vi "closed_loop_arbitrary_binary_stim.vi"() -> ()   [LabVIEW 2014]
uses:
  <vilib>/vision/Measure.llb/Straight Edge Options.ctl
  <vilib>/vision/Measure.llb/Straight Edge Process.ctl
  <vilib>/Platform/TimedLoop/XDataNode/timing_clust.ctl
  <vilib>/Platform/TimedLoop/XDataNode/nitl_modes.ctl
  <vilib>/Platform/TimedLoop/XDataNode/wakeup.ctl
  <vilib>/vision/Measure.llb/Edge Options.ctl
  <vilib>/vision/Measure.llb/Edge Polarity.ctl
  <vilib>/DAQmx/create/channels.llb/DAQmx Create Channel (DO-Digital Output).vi
  <vilib>/DAQmx/write.llb/DAQmx Write (Digital Bool 1Line 1Point).vi
  <vilib>/gmath/statdist.llb/Uniform (Discrete) Random.vi
  <vilib>/DAQmx/create/channels.llb/DAQmx Create Channel (AO-Voltage-Basic).vi
  <vilib>/Platform/TimedLoop/TimeConversion.llb/rt-rel-time-to-milliseconds.vi
  <vilib>/DAQmx/write.llb/DAQmx Write (Analog DBL 1Chan 1Samp).vi
  <vilib>/DAQmx/create/channels.llb/DAQmx Create Channel (DI-Digital Input).vi
  <vilib>/DAQmx/read.llb/DAQmx Read (Digital Bool 1Line 1Point).vi
  <vilib>/platform/TimedLoop/XDataNode/XDataNode.xnode
  <vilib>/vision/driver/NI_Vision_Acquisition_Software.lvlib
  <vilib>/Platform/TimedLoop/XDataNode/XDNodeRunTimeDep.lvlib
  <vilib>/vision/NI_Vision_Development_Module.lvlib
  <vilib>/gmath/NI_Gmath.lvlib
panel:
  out "Slide 5":dbl(slide) scale=0.0..1.0
  out "Stim 4":i32
  in  "Stimulus Folder":path=path "C:/Users/nagellab/Documents/MATLAB/wind_pulses"
  in  "Stimulus Duration (s)":dbl=80.0
  out "Light History":i16(graph)
  out "Wind History":i16(graph)
  in  "Initial Orientation (for each trial)":dbl
  out "Light":bool=TRUE
  in  "Light Intensity (V)":dbl=3.9 format="%#_13g"
  in  "Wind Intensity (V)":dbl=3.1 format="%#_13g"
  out "Wind":bool=TRUE
  out "H0":dbl
  out "Slide 4":dbl(slide) scale=0.0..1.0
  out "Slide 3":dbl(slide) scale=0.0..1.0
  out "Slide 2":dbl(slide) scale=0.0..1.0
  out "Stim 3":i32
  out "Stim 2":i32
  out "Stim 1":i32
  in  "Reversed Tether?":bool=TRUE
  in  "R options":T1={"Number of Lines"=1, "Type"=enum."Best Edge Projection", "Min. Score"=10.0, "Max. Score"=1000.0, "Orientation"=-135.0, "Angle Range"=45.0, "Angle Tolerance"=1.0, "Step Size"=3, "Min. SNR (db)"=0.0, "Min. Points (%)"=25.0, "Hough Iterations"=3} {"Min. Points (%)" min=0.0 max=100.0; "Min. SNR (db)" min=0.0; "Max. Score" min=0.0 max=1024.0; "Min. Score" min=0.0 max=1024.0 step=1.0}
  in  "L options":T1={"Number of Lines"=1, "Type"=enum."Best Edge Projection", "Min. Score"=10.0, "Max. Score"=1000.0, "Orientation"=135.0, "Angle Range"=45.0, "Angle Tolerance"=1.0, "Step Size"=3, "Min. SNR (db)"=0.0, "Min. Points (%)"=25.0, "Hough Iterations"=3} {"Min. Points (%)" min=0.0 max=100.0; "Min. SNR (db)" min=0.0; "Max. Score" min=0.0 max=1024.0; "Min. Score" min=0.0 max=1024.0 step=1.0}
  out "Slide":dbl(slide) scale=0.0..1.0
  out "Motor Error":bool
  in  "Max steps/sample":dbl=6.0
  in  "Step Rate (Hz)":dbl=500.0
  out "Heading (deg)":dbl(graph)
  out "H":dbl format="%.4f"
  out "X (steps/sample)":dbl
  in  "Geneotype":string="w+ Canton-S"
  in  "Starvation Time (hrs)":string="1"
  in  "Age (DSE)":string="4"
  out "Trial End":bool
  in  "Trial Duration (s)":dbl=80.0
  out "Trial":i32 format="%#.3f"
  in  "Number of Trials":i32=12
  in  "Experiment name":string="E1"
  in  "Fly ID":string
  in  "L-R WBA Offset (deg)":dbl format="%#_13g"
  in  "deltaWBA Gain (g, unitless)":dbl=0.04 format="%.4f"
  out "L-R WBA":dbl
  out "deltaWBA":dbl format="%.4f"
  out "Scaled deltaWBA (deg)":dbl(graph)
  out "R WBA":dbl
  out "L WBA":dbl
  out "Image":T3(plugin-control)
  in  "Image Threshold":cluster{"Lower value":sgl, "Upper value":sgl}={"Lower value"=130.0, "Upper value"=255.0} {"Upper value" format="%.2f"; "Lower value" format="%.2f"}
  in  "Data Rate (Hz)":dbl=50.0
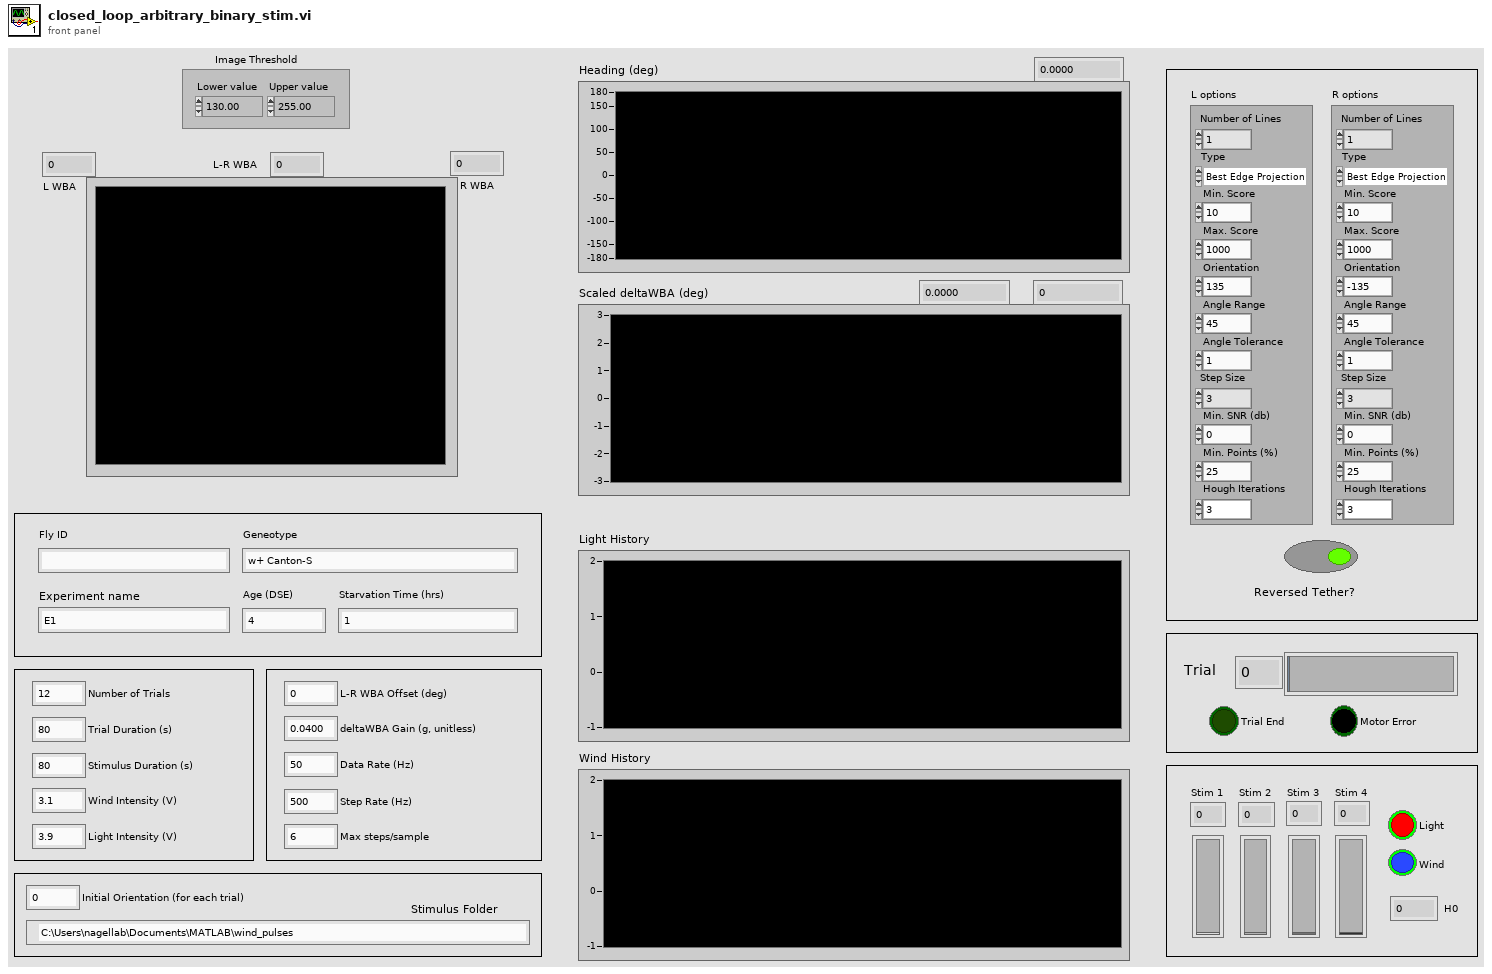
[diagram p1: front panel]
types:
  T1 = typedef "Straight Edge Options.ctl" = cluster{"Number of Lines":i32, "Type":T2, "Min. Score":dbl, "Max. Score":dbl, "Orientation":dbl, "Angle Range":dbl, "Angle Tolerance":dbl, "Step Size":u32, "Min. SNR (db)":dbl, "Min. Points (%)":dbl, "Hough Iterations":i32}
  T2 = typedef "Straight Edge Process.ctl" = enum32{"First Edge Rake", "Best Edge Rake", "Hough Edge Rake", "First Edge Projection", "Best Edge Projection"}
  T3 = typedef "IMAQ Image.ctl" = refnum<image>
  T4 = enum16{"open", "replace", "create", "open or create", "replace or create", "replace or create with confirmation"}
  T5 = typedef "IMAQdx.ctl" = refnum<k21>
  T6 = typedef "IMAQ Rectangle" = cluster{"Left":i32, "Top":i32, "Right":i32, "Bottom":i32, "Rotation":dbl}
  T7 = typedef "ROI Descriptor" = cluster{"Global Rectangle":i32[], "Contours":cluster{"ID":enum32{"External", "Internal"}, "Type":u32, "Coordinates":i32[]}[]}
  T8 = enum16{"big-endian, network order", "native, host order", "little-endian"}
  T9 = typedef "XDNodeRunTimeDep.lvlib/timing_clust.ctl" = cluster{"Expected End [f-1]":u64, "Actual End [f-1]":u64, "Finished Late? [f-1]":bool, "Expected End [i-1]":u64, "Actual End [i-1]":u64, "Finished Late? [i-1]":bool, "Expected Start [i]":u64, "Actual Start [i]":u64, "Expected Start [f]":u64, "Actual Start [f]":u64, "Source Name":string, "Structure Name":string, "Period":i64, "Deadline":i64, "Offset":i64, "Start":i64, "Priority":i32, "Timeout":i32, "Mode":T10, "Wakeup Reason":T11, "Error":errorcluster, "Source Type":string, "Secondary Source Type":string, "Global End Time":u64, "Global Start Time":u64, "Frame Duration":u64, "Iteration Duration":u64, "Assigned CPU":i32, "I/O Scan Engine Mode":u32}
  T10 = typedef "XDNodeRunTimeDep.lvlib/nitl_modes.ctl" = enum32{"No Change", "Process missed periods, maintain original phase", "Discard missed periods, maintain original phase", "Process missed periods, ignore original phase", "Discard missed periods, ignore original phase"}
  T11 = typedef "XDNodeRunTimeDep.lvlib/wakeup.ctl" = enum32{"Normal", "Aborted", "Asynchronous wakeup", "Timing source error", "Timed loop error", "Timeout"}
  T12 = cluster{"y":i32, "y":i32, "y":i32, "y":i32, "y":i32, "y":i32}
  T13 = typedef "Edge Options.ctl" = cluster{"Edge Polarity":T14, "Kernel Size":u32, "Width":u32, "Minimum Edge Strength":sgl, "Interpolation Type":enum32{"Zero Order", "Bilinear", "Quadratic", "Cubic", "Bilinear Fixed"}, "Data Processing Method":enum32{"Average", "Median"}}
  T14 = typedef "Edge Polarity.ctl" = u32
  T15 = cluster{"Search Direction":u32, "Edge Options":T13, "Show Search Area":bool, "Show Search Lines":bool, "Show Edges Found":bool, "Show Result":bool, "Search Area Color":u32, "Search Lines Color":u32, "Edge Locations Color":u32, "Result Color":u32, "Overlay Group Name":string}
  T16 = cluster{"Point1 (Pixels)":cluster{"X":sgl, "Y":sgl}, "Point2 (Pixels)":cluster{"X":sgl, "Y":sgl}, "Point1 (Real-World)":cluster{"X":sgl, "Y":sgl}, "Point2 (Real-World)":cluster{"X":sgl, "Y":sgl}, "Angle (Pixel)":dbl, "Angle (Real-World)":dbl, "Score":dbl, "Straightness":dbl, "Average SNR (db)":dbl, "Calibration Valid":bool}[]
  T17 = cluster{"Straight Edges[0]":cluster{"Point1 (Pixels)":cluster{"X":sgl, "Y":sgl}, "Point2 (Pixels)":cluster{"X":sgl, "Y":sgl}, "Point1 (Real-World)":cluster{"X":sgl, "Y":sgl}, "Point2 (Real-World)":cluster{"X":sgl, "Y":sgl}, "Angle (Pixel)":dbl, "Angle (Real-World)":dbl, "Score":dbl, "Straightness":dbl, "Average SNR (db)":dbl, "Calibration Valid":bool}, "Straight Edges[1]":cluster{"Point1 (Pixels)":cluster{"X":sgl, "Y":sgl}, "Point2 (Pixels)":cluster{"X":sgl, "Y":sgl}, "Point1 (Real-World)":cluster{"X":sgl, "Y":sgl}, "Point2 (Real-World)":cluster{"X":sgl, "Y":sgl}, "Angle (Pixel)":dbl, "Angle (Real-World)":dbl, "Score":dbl, "Straightness":dbl, "Average SNR (db)":dbl, "Calibration Valid":bool}, "Straight Edges[2]":cluster{"Point1 (Pixels)":cluster{"X":sgl, "Y":sgl}, "Point2 (Pixels)":cluster{"X":sgl, "Y":sgl}, "Point1 (Real-World)":cluster{"X":sgl, "Y":sgl}, "Point2 (Real-World)":cluster{"X":sgl, "Y":sgl}, "Angle (Pixel)":dbl, "Angle (Real-World)":dbl, "Score":dbl, "Straightness":dbl, "Average SNR (db)":dbl, "Calibration Valid":bool}, "Straight Edges[3]":cluster{"Point1 (Pixels)":cluster{"X":sgl, "Y":sgl}, "Point2 (Pixels)":cluster{"X":sgl, "Y":sgl}, "Point1 (Real-World)":cluster{"X":sgl, "Y":sgl}, "Point2 (Real-World)":cluster{"X":sgl, "Y":sgl}, "Angle (Pixel)":dbl, "Angle (Real-World)":dbl, "Score":dbl, "Straightness":dbl, "Average SNR (db)":dbl, "Calibration Valid":bool}, "Straight Edges[4]":cluster{"Point1 (Pixels)":cluster{"X":sgl, "Y":sgl}, "Point2 (Pixels)":cluster{"X":sgl, "Y":sgl}, "Point1 (Real-World)":cluster{"X":sgl, "Y":sgl}, "Point2 (Real-World)":cluster{"X":sgl, "Y":sgl}, "Angle (Pixel)":dbl, "Angle (Real-World)":dbl, "Score":dbl, "Straightness":dbl, "Average SNR (db)":dbl, "Calibration Valid":bool}, "Straight Edges[5]":cluster{"Point1 (Pixels)":cluster{"X":sgl, "Y":sgl}, "Point2 (Pixels)":cluster{"X":sgl, "Y":sgl}, "Point1 (Real-World)":cluster{"X":sgl, "Y":sgl}, "Point2 (Real-World)":cluster{"X":sgl, "Y":sgl}, "Angle (Pixel)":dbl, "Angle (Real-World)":dbl, "Score":dbl, "Straightness":dbl, "Average SNR (db)":dbl, "Calibration Valid":bool}, "Straight Edges[6]":cluster{"Point1 (Pixels)":cluster{"X":sgl, "Y":sgl}, "Point2 (Pixels)":cluster{"X":sgl, "Y":sgl}, "Point1 (Real-World)":cluster{"X":sgl, "Y":sgl}, "Point2 (Real-World)":cluster{"X":sgl, "Y":sgl}, "Angle (Pixel)":dbl, "Angle (Real-World)":dbl, "Score":dbl, "Straightness":dbl, "Average SNR (db)":dbl, "Calibration Valid":bool}, "Straight Edges[7]":cluster{"Point1 (Pixels)":cluster{"X":sgl, "Y":sgl}, "Point2 (Pixels)":cluster{"X":sgl, "Y":sgl}, "Point1 (Real-World)":cluster{"X":sgl, "Y":sgl}, "Point2 (Real-World)":cluster{"X":sgl, "Y":sgl}, "Angle (Pixel)":dbl, "Angle (Real-World)":dbl, "Score":dbl, "Straightness":dbl, "Average SNR (db)":dbl, "Calibration Valid":bool}, "Straight Edges[8]":cluster{"Point1 (Pixels)":cluster{"X":sgl, "Y":sgl}, "Point2 (Pixels)":cluster{"X":sgl, "Y":sgl}, "Point1 (Real-World)":cluster{"X":sgl, "Y":sgl}, "Point2 (Real-World)":cluster{"X":sgl, "Y":sgl}, "Angle (Pixel)":dbl, "Angle (Real-World)":dbl, "Score":dbl, "Straightness":dbl, "Average SNR (db)":dbl, "Calibration Valid":bool}}
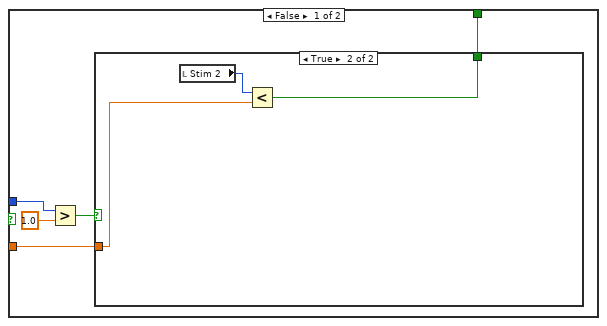
[diagram p2: hidden frame]
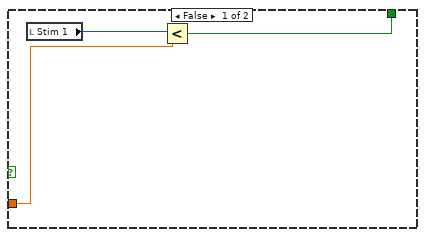
[diagram p3: hidden frame]
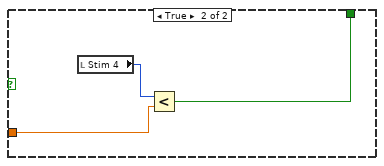
[diagram p4: hidden frame]
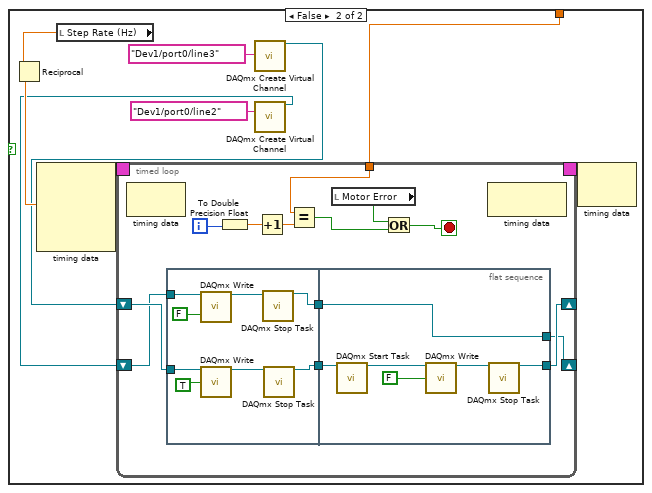
[diagram p6: hidden frame]
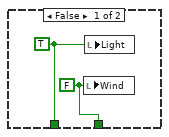
[diagram p8: hidden frame]
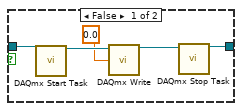
[diagram p9: hidden frame]
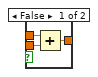
[diagram p10: hidden frame]
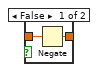
[diagram p11: hidden frame]
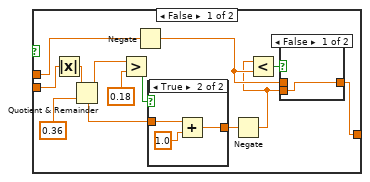
[diagram p12: hidden frame]
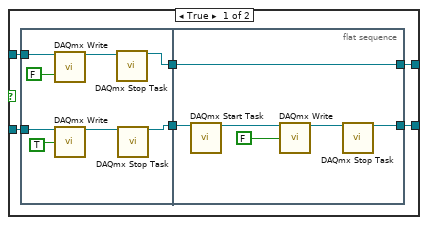
[diagram p18: hidden frame]
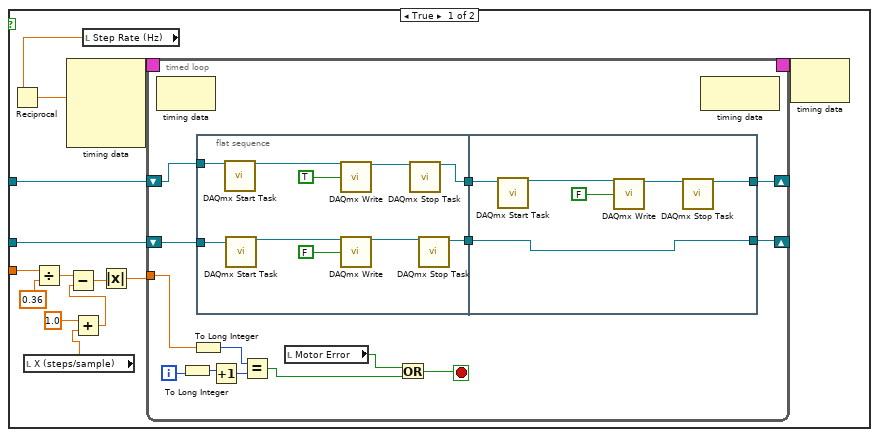
[diagram p20: hidden frame]
diagram:
  w77 = "."
  w79 = "."
  n1 = local read "Wind Intensity (V)"() -> (w24:dbl)
  n2 = local read "Data Rate (Hz)"() -> (w58:dbl)
  n3 = local read "Trial Duration (s)"() -> (w63:dbl)
  n4 = local read "Number of Trials"() -> (w65:i32)
  n5 = local read "Light Intensity (V)"() -> (w22:dbl)
  n6 = local read "deltaWBA Gain (g, unitless)"() -> (w57:dbl)
  n7 = local read "Max steps/sample"() -> (w55:dbl)
  n8 = local read "Step Rate (Hz)"() -> (w56:dbl)
  n9 = local read "Reversed Tether?"() -> (w44:bool)
  n10 = local read "Stimulus Duration (s)"() -> (w13:dbl)
  n11 = Boolean To (0,1)(Boolean=w44) -> (0, 1=w45:i16)
  n12 = To Double Precision Float(number=w45) -> (double precision float=w43:dbl)
  n13 = Number To Fractional String(number=w22, precision (6)=i16 3) -> (F-format string=w20:string)  [unwired: 2 in]
  n14 = Number To Fractional String(number=w65, precision (6)=i16 0) -> (F-format string=w49:string)  [unwired: 2 in]
  n15 = Number To Fractional String(number=w63, precision (6)=i16 0) -> (F-format string=w48:string)  [unwired: 2 in]
  n16 = Number To Fractional String(number=w24, precision (6)=i16 3) -> (F-format string=w21:string)  [unwired: 2 in]
  n17 = Number To Fractional String(number=w58, precision (6)=i16 0) -> (F-format string=w19:string)  [unwired: 2 in]
  n18 = Number To Fractional String(number=w56, precision (6)=i16 0) -> (F-format string=w18:string)  [unwired: 2 in]
  n19 = Number To Fractional String(number=w55, precision (6)=i16 0) -> (F-format string=w17:string)  [unwired: 2 in]
  n20 = Number To Fractional String(number=w57, precision (6)=i16 3) -> (F-format string=w16:string)  [unwired: 2 in]
  n21 = Number To Fractional String(number=w43, precision (6)=i16 0) -> (F-format string=w15:string)  [unwired: 2 in]
  n22 = Number To Fractional String(number=w13, precision (6)=i16 0) -> (F-format string=w12:string)  [unwired: 2 in]
  n23 = Get Date/Time In Seconds() -> (seconds since 1Jan1904=w85:timestamp)
  n24 = Get Date/Time In Seconds() -> (seconds since 1Jan1904=w81:timestamp)
  n25 = Get Date/Time In Seconds() -> (seconds since 1Jan1904=w83:timestamp)
  n26 = call <vilib>:"Space Constant.vi"() -> ("String"=w87:string)
  n27 = Format Date/Time String(time format string (%c)="%d", seconds (now)=w85) -> (date/time string=w76:string)  [unwired: 1 in]
  n28 = Format Date/Time String(time format string (%c)="%m", seconds (now)=w83) -> (date/time string=w78:string)  [unwired: 1 in]
  n29 = Format Date/Time String(time format string (%c)="%Y", seconds (now)=w81) -> (date/time string=w80:string)  [unwired: 1 in]
  n30 = Concatenate Strings(w80, w79, w78, w77, w76) -> (w54:string)
  n31 = Concatenate Strings(w80, w79, w78, w77, w76, w87, "fly_", "Fly ID", "\\") -> (w91:string)
  n32 = String To Path(string=w91) -> (path=w90:path)
  n33 = Build Path(base path=path "E:/TAC DATA ARCHIVE/NewRig/labview/WindPulses", name or relative path=w90) -> (appended path=w95:path)
  n34 = call <vilib>:"IMAQdx Open Camera.vi"("Session In"=refnum<k21> "cam8" ("Camera Name")) -> ("Session Out"=w117:T5)  [unwired: 2 in, 8 out]
  n35 = call <vilib>:"Check if File or Folder Exists.vi"("path"=w95) -> ("file or folder exists?"=w93:bool, "dup path"=w94:path)  [unwired: 8 in, 1 out]
  n36 = call <vilib>:"IMAQdx Configure Grab.vi"("Session In"=w117) -> ("Session Out"=w115:T5)  [unwired: 1 in, 9 out]
  n37 = case shown="False" w93 {
    tunnel: w94 -> [w119 w120]
    tunnel: [w118 w120] -> w99
    frame False {
      n38 = Create Folder(path (use dialog)=w119) -> (created path=w118:path)  [unwired: 2 in, 2 out]
    }
    frame True {
    }
  }
  n39 = call "IMAQ Create"("Image Name"="ROIR") -> ("New Image"=w114:T3)  [unwired: 3 in, 2 out]
  n40 = Concatenate Strings("Experiment name", "\\") -> (w67:string)
  n41 = call <vilib>:"IMAQdx Grab.vi"("Image In"=w114, "Session In"=w115) -> ("Image Out"=w113:T3, "Session Out"=w104:T5)  [unwired: 2 in, 6 out]
  n42 = String To Path(string=w67) -> (path=w96:path)
  n43 = call "IMAQ Select Rectangle"("Prompt"="Select RIGHT ROI for wing angle detection", "Image In"=w113) -> ("Rectangle"=w105:T6)  [unwired: 6 in, 3 out]
  n44 = Build Path(base path=w99, name or relative path=w96) -> (appended path=w100:path)
  n45 = call "IMAQ Convert Rectangle to ROI"("Rectangle"=w105) -> ("ROI Descriptor"=w103:T7)  [unwired: 8 in, 1 out]
  n46 = call <vilib>:"Check if File or Folder Exists.vi"("path"=w100) -> ("file or folder exists?"=w97:bool, "dup path"=w98:path)  [unwired: 8 in, 1 out]
  n47 = call "IMAQ Create"("Image Name"="ROIL") -> ("New Image"=w109:T3)  [unwired: 3 in, 2 out]
  n48 = case shown="False" w97 {
    tunnel: w98 -> [w122 w123]
    tunnel: [w121 w123] -> w5
    frame False {
      n49 = Create Folder(path (use dialog)=w122) -> (created path=w121:path)  [unwired: 2 in, 2 out]
    }
    frame True {
    }
  }
  n50 = call <vilib>:"IMAQdx Grab.vi"("Image In"=w109, "Session In"=w104) -> ("Image Out"=w108:T3, "Session Out"=w102:T5)  [unwired: 2 in, 6 out]
  n51 = String To Path(string="experiment_information") -> (path=w75:path)
  n52 = call "IMAQ Select Rectangle"("Prompt"="Select LEFT ROI for wing angle detection", "Image In"=w108) -> ("Rectangle"=w110:T6)  [unwired: 6 in, 3 out]
  n53 = Build Path(base path=w5, name or relative path=w75) -> (appended path=w72:path)
  n54 = String To Path(string="initial_orientations") -> (path=w34:path)
  n55 = String To Path(string="stimulus_ID") -> (path=w10:path)
  n56 = call "IMAQ Convert Rectangle to ROI"("Rectangle"=w110) -> ("ROI Descriptor"=w101:T7)  [unwired: 8 in, 1 out]
  n57 = Build Path(base path=w5, name or relative path=w34) -> (appended path=w31:path)
  n58 = Build Path(base path=w5, name or relative path=w10) -> (appended path=w7:path)
  n59 = Open/Create/Replace File(file path (use dialog)=w72, operation (0:open)=T4."create", access (0:read/write)=enum16{"read/write", "read-only", "write-only"}."write-only") -> (refnum out=w70:refnum<file>)  [unwired: 3 in, 2 out]
  n60 = Open/Create/Replace File(file path (use dialog)=w31, operation (0:open)=T4."create", access (0:read/write)=enum16{"read/write", "read-only", "write-only"}."write-only") -> (refnum out=w29:refnum<file>)  [unwired: 3 in, 2 out]
  n61 = Open/Create/Replace File(file path (use dialog)=w7, operation (0:open)=T4."create", access (0:read/write)=enum16{"read/write", "read-only", "write-only"}."write-only") -> (refnum out=w3:refnum<file>)  [unwired: 3 in, 2 out]
  n62 = Build Array(w54, "Fly ID", "Experiment name", "Age (DSE)", "Starvation Time (hrs)", w49, w48, w21, w20, w19, w18, w17, w16, w15, w12, "Geneotype") -> (w47:string[])
  n63 = Write to Text File(file (use dialog)=w70, text=w47) -> (refnum out=w69:refnum<file>)  [unwired: 2 in, 2 out]
  n64 = Close File(refnum=w69) -> ()  [unwired: 1 in, 2 out]
  n65 = flat-sequence {
    tunnel: w5 -> [w127]
    tunnel: w101 -> [w128]
    tunnel: w102 -> [w129]
    tunnel: w103 -> [w130]
    tunnel: [w130] -> w42
    tunnel: [w129] -> w40
    tunnel: [w128] -> w38
    tunnel: [w127] -> w36
    tunnel: w29 -> [w125]
    tunnel: [w125] -> w27
    tunnel: [w124] -> w4
    tunnel: w3 -> [w124]
    tunnel: w42 -> [w136]
    tunnel: [w136] -> w41
    tunnel: w40 -> [w135]
    tunnel: [w135] -> w39
    tunnel: w38 -> [w134]
    tunnel: [w134] -> w37
    tunnel: w36 -> [w133]
    tunnel: [w133] -> w35
    tunnel: [w132] -> w28
    tunnel: w27 -> [w132]
    tunnel: w4 -> [w131]
    tunnel: [w131] -> w2
    tunnel: w41 -> [w151]
    tunnel: w39 -> [w150]
    tunnel: w37 -> [w149]
    tunnel: w35 -> [w148]
    tunnel: w28 -> [w142]
    tunnel: [w141] -> w26
    tunnel: w2 -> [w138]
    tunnel: [w137] -> w1
    tunnel: w26 -> [w1087]
    tunnel: w1 -> [w1081]
    frame #0 {
      n66 = One Button Dialog(message="Ensure the stage is at 0 degrees.") -> ()  [unwired: 1 in, 1 out]
    }
    frame #1 {
    }
    frame #2 {
      n67 = for {
        N: "Number of Trials" -> [_]
        tunnel: w151 -> [w233]
        tunnel: w150 -> [w232]
        tunnel: w149 -> [w231]
        tunnel: w148 -> [w230]
        shift-right: [w209] -> _
        shift-left: 0 ("y") -> [w204]
        shift-right: [w208] -> _
        shift-left: 0 ("y") -> [w202]
        shift-right: [w207] -> _
        shift-left: 0 ("y") -> [w200]
        shift-right: [w206] -> _
        shift-left: 0 ("y") -> [w154]
        shift-right: [w160] -> w141
        shift-left: w142 -> [w178]
        shift-right: [w170] -> _
        shift-left: 0 ("y") -> [w174]
        shift-right: [w171] -> _
        shift-left: 0 ("y") -> [w175]
        shift-right: [w156] -> w137
        shift-left: w138 -> [w159]
        i -> [w227]
        n68 = local read "Number of Trials"() -> (w205:i32)
        n69 = local read "Number of Trials"() -> (w218:i32)
        n70 = Divide(x=w205, y=4) -> (x/y=w152:dbl)
        n71 = Divide(x=w154, y=w152) -> (x/y=→"Slide 5":dbl)
        n72 = Divide(x=w204, y=w152) -> (x/y=→"Slide 2":dbl)
        n73 = Divide(x=w200, y=w152) -> (x/y=→"Slide 4":dbl)
        n74 = Divide(x=w202, y=w152) -> (x/y=→"Slide 3":dbl)
        n75 = flat-sequence {
          tunnel: w217 -> [w257]
          tunnel: w230 -> [w258]
          tunnel: w231 -> [w259]
          tunnel: w232 -> [w260]
          tunnel: w233 -> [w261]
          tunnel: [w261] -> w199
          tunnel: [w260] -> w197
          tunnel: [w259] -> w195
          tunnel: [w258] -> w193
          tunnel: [w257] -> w191
          tunnel: [w249] -> w189
          tunnel: w200 -> [w246]
          tunnel: w154 -> [w245]
          tunnel: w202 -> [w247]
          tunnel: w204 -> [w248]
          tunnel: w152 -> [w244]
          tunnel: [w248] -> w187
          tunnel: [w247] -> w186
          tunnel: [w246] -> w185
          tunnel: [w245] -> w184
          tunnel: w178 -> [w243]
          tunnel: [w243] -> w177
          tunnel: w174 -> [w242]
          tunnel: w175 -> [w241]
          tunnel: [w242] -> w173
          tunnel: [w241] -> w172
          tunnel: w159 -> [w239]
          tunnel: [w239] -> w158
          tunnel: w199 -> [w317]
          tunnel: [w317] -> w198
          tunnel: w197 -> [w316]
          tunnel: [w316] -> w196
          tunnel: w195 -> [w315]
          tunnel: [w315] -> w194
          tunnel: w193 -> [w314]
          tunnel: [w314] -> w192
          tunnel: w191 -> [w313]
          tunnel: [w313] -> w190
          tunnel: w189 -> [w294]
          tunnel: [w312] -> w188
          tunnel: w187 -> [w311]
          tunnel: w186 -> [w310]
          tunnel: w185 -> [w309]
          tunnel: w184 -> [w308]
          tunnel: [w306] -> w183
          tunnel: [w294] -> w182
          tunnel: w177 -> [w305]
          tunnel: [w304] -> w176
          tunnel: w173 -> [w302]
          tunnel: w172 -> [w301]
          tunnel: [w298] -> w168
          tunnel: [w297] -> w167
          tunnel: w158 -> [w296]
          tunnel: [w293] -> w157
          tunnel: [w452] -> w238
          tunnel: [w451] -> w237
          tunnel: [w450] -> w236
          tunnel: [w419] -> w235
          tunnel: w198 -> [w452]
          tunnel: w196 -> [w451]
          tunnel: w194 -> [w450]
          tunnel: w192 -> [w356]
          tunnel: w190 -> [w357]
          tunnel: [w418] -> w226
          tunnel: [w417] -> w223
          tunnel: [w396] -> w222
          tunnel: [w395] -> w221
          tunnel: [w394] -> w215
          tunnel: w188 -> [w393]
          tunnel: [w393] -> w212
          tunnel: w183 -> [w392]
          tunnel: w182 -> [w380]
          tunnel: [w380] -> w181
          tunnel: w176 -> [w353]
          tunnel: w168 -> [w378]
          tunnel: w167 -> [w379]
          tunnel: [w379] -> w166
          tunnel: [w378] -> w165
          tunnel: [w355] -> w164
          tunnel: [w354] -> w163
          tunnel: [w353] -> w160
          tunnel: [w352] -> w156
          tunnel: w157 -> [w352]
          tunnel: w238 -> [w585]
          tunnel: w237 -> [w584]
          tunnel: w236 -> [w583]
          tunnel: w235 -> [w582]
          tunnel: [w581] -> w234
          tunnel: [w580] -> w229
          tunnel: [w579] -> w228
          tunnel: w226 -> [w578]
          tunnel: [w577] -> w225
          tunnel: [w576] -> w224
          tunnel: w223 -> [w575]
          tunnel: w222 -> [w574]
          tunnel: w221 -> [w573]
          tunnel: [w572] -> w220
          tunnel: [w571] -> w219
          tunnel: w215 -> [w564]
          tunnel: [w561] -> w214
          tunnel: [w558] -> w213
          tunnel: w212 -> [w557]
          tunnel: [w557] -> w211
          tunnel: w181 -> [w556]
          tunnel: [w556] -> w180
          tunnel: w166 -> [w554]
          tunnel: w165 -> [w555]
          tunnel: w164 -> [w552]
          tunnel: w163 -> [w551]
          tunnel: [w550] -> w162
          tunnel: [w549] -> w161
          tunnel: w234 -> [w848]
          tunnel: w229 -> [w851]
          tunnel: w228 -> [w850]
          tunnel: w225 -> [w849]
          tunnel: w224 -> [w847]
          tunnel: w220 -> [w846]
          tunnel: w219 -> [w845]
          tunnel: w214 -> [w841]
          tunnel: w213 -> [w835]
          tunnel: w211 -> [w833]
          tunnel: [w833] -> w210
          tunnel: w180 -> [w830]
          tunnel: [w830] -> w179
          tunnel: w162 -> [w829]
          tunnel: w161 -> [w828]
          tunnel: w210 -> [w973]
          tunnel: [w972] -> w209
          tunnel: [w971] -> w208
          tunnel: [w970] -> w207
          tunnel: [w969] -> w206
          tunnel: w179 -> [w963]
          tunnel: [w959] -> w170
          tunnel: [w958] -> w171
          frame #0 {
            n76 = while {
              tunnel: w244 -> [w263]
              tunnel: [w264] -> w249
              stop <- w262 stop-if-true
              n77 = call-poly <vilib>:"Discrete Random.vi"("n"=4, "samples"=1) -> ("uniform (discrete) random data"=w267:i32[])  [unwired: 8 in, 1 out]
              n78 = Index Array(array=w267, index=0) -> (element=w264:i32)
              n79 = Greater?(x=w264, y=2.0) -> (0:w265:bool)
              n80 = case shown="True" w265 {
                tunnel: w264 -> [w271 w285]
                tunnel: w263 -> [w273 w283]
                tunnel: [w272 w282] -> w262
                frame False {
                  n81 = Greater?(x=w271, y=1.0) -> (0:w274:bool)
                  n82 = case shown="True" w274 {
                    tunnel: w273 -> [w277 w280]
                    tunnel: [w276 w279] -> w272
                    frame False {
                      n83 = local read "Stim 1"() -> (w278:i32)
                      n84 = Less?(x=w278, y=w277) -> (x < y?=w276:bool)
                    }
                    frame True {
                      n85 = local read "Stim 2"() -> (w281:i32)
                      n86 = Less?(x=w281, y=w280) -> (x < y?=w279:bool)
                    }
                  }
                }
                frame True {
                  n87 = Greater?(x=w285, y=3.0) -> (0:w284:bool)
                  n88 = case shown="False" w284 {
                    tunnel: w283 -> [w289 w292]
                    tunnel: [w287 w290] -> w282
                    frame False {
                      n89 = local read "Stim 3"() -> (w288:i32)
                      n90 = Less?(x=w288, y=w289) -> (x < y?=w287:bool)
                    }
                    frame True {
                      n91 = local read "Stim 4"() -> (w291:i32)
                      n92 = Less?(x=w291, y=w292) -> (x < y?=w290:bool)
                    }
                  }
                }
              }
            }
            n93 = call-poly <vilib>:"DAQmx Create Virtual Channel.vi"("lines"=tag "Dev1/port0/line0") -> ("task out"=w255:refnum<k21>)  [unwired: 13 in, 1 out]
            n94 = call <vilib>:"DAQmx Start Task.vi"("task/channels in"=w255) -> ("task out"=w254:refnum<k21>)  [unwired: 13 in, 1 out]
            n95 = call-poly <vilib>:"DAQmx Write.vi"("task/channels in"=w254, "data"=FALSE) -> ("task out"=w253:refnum<k21>)  [unwired: 11 in, 2 out]
            n96 = call <vilib>:"DAQmx Stop Task.vi"("task/channels in"=w253) -> ()  [unwired: 13 in, 2 out]
            n97 = local write "Motor Error"(FALSE ("Trial End")) -> ()
            n98 = local write "Trial End"(FALSE ("Trial End")) -> ()
            "H0" <- "Initial Orientation (for each trial)"
          }
          frame #1 {
            n99 = flat-sequence {
              tunnel: [w338] -> w298
              tunnel: [w336] -> w300
              tunnel: w294 -> [w335]
              tunnel: w300 -> [w351]
              frame #0 {
                n100 = Number To Fractional String(number=w335, precision (6)=i16 0) -> (F-format string=w349:string)  [unwired: 2 in]
                n101 = Concatenate Strings("stim" ("string"), w349, "light\\" ("string")) -> (w346:string)
                n102 = Build Path(base path="Stimulus Folder", name or relative path=w346) -> (appended path=w344:path)
                n103 = Open/Create/Replace File(file path (use dialog)=w344, operation (0:open)=T4."open", access (0:read/write)=enum16{"read/write", "read-only", "write-only"}."read-only") -> (refnum out=w341:refnum<file>)  [unwired: 3 in, 2 out]
                n104 = Read from Binary File(5:0.0 ("element"), 9:T8."big-endian, network order" ("byte order (0:big-endian, network order)"), 10:-1 ("count (1)"), 11:w341) -> (2:w338:dbl[], 3:w336:refnum<file>)  [unwired: 2 in, 2 out]
              }
              frame #1 {
                n105 = Close File(refnum=w351) -> ()  [unwired: 1 in, 2 out]
              }
            }
            n106 = flat-sequence {
              tunnel: [w322] -> w297
              tunnel: [w320] -> w299
              tunnel: w294 -> [w319]
              tunnel: w299 -> [w334]
              frame #0 {
                n107 = Number To Fractional String(number=w319, precision (6)=i16 0) -> (F-format string=w332:string)  [unwired: 2 in]
                n108 = local read "Stimulus Folder"() -> (w318:path)
                n109 = Concatenate Strings("stim" ("string"), w332, "wind\\" ("string")) -> (w329:string)
                n110 = Build Path(base path=w318, name or relative path=w329) -> (appended path=w328:path)
                n111 = Open/Create/Replace File(file path (use dialog)=w328, operation (0:open)=T4."open", access (0:read/write)=enum16{"read/write", "read-only", "write-only"}."read-only") -> (refnum out=w325:refnum<file>)  [unwired: 3 in, 2 out]
                n112 = Read from Binary File(5:0.0 ("element"), 9:T8."big-endian, network order" ("byte order (0:big-endian, network order)"), 10:-1 ("count (1)"), 11:w325) -> (2:w322:dbl[], 3:w320:refnum<file>)  [unwired: 2 in, 2 out]
              }
              frame #1 {
                n113 = Close File(refnum=w334) -> ()  [unwired: 1 in, 2 out]
              }
            }
            n114 = local read "H0"() -> (w303:dbl)
            n115 = To Double Precision Float(number=w294) -> (double precision float=w295:dbl)
            n116 = Write to Binary File(file (use dialog)=w296, data=w295) -> (refnum out=w293:refnum<file>)  [unwired: 4 in, 2 out]
            n117 = Write to Binary File(file (use dialog)=w305, data=w303) -> (refnum out=w304:refnum<file>)  [unwired: 4 in, 2 out]
            n118 = call-poly <vilib>:"DAQmx Create Virtual Channel.vi"("physical channels"=tag "Dev1/ao1") -> ("task out"=w306:refnum<k21>)  [unwired: 13 in, 1 out]
            n119 = Bundle("y"=w311, "y"=w310, "y"=w309, "y"=w308, "y"=w302, "y"=w301) -> (w312:T12)  [unwired: 1 in]
          }
          frame #2 {
            n120 = flat-sequence {
              tunnel: ["Wind Intensity (V)"] -> w391
              tunnel: w392 -> [w544]
              tunnel: w391 -> [w542]
              frame #0 {
              }
              frame #1 {
                n121 = Greater Than 0?(x=w542) -> (x > 0?=w543:bool)
                n122 = case shown="True" w543 {
                  tunnel: w544 -> [_ w548]
                  tunnel: w542 -> [_ w545]
                  frame False {
                  }
                  frame True {
                    n123 = call <vilib>:"DAQmx Start Task.vi"("task/channels in"=w548) -> ("task out"=w547:refnum<k21>)  [unwired: 13 in, 1 out]
                    n124 = call-poly <vilib>:"DAQmx Write.vi"("task/channels in"=w547, "data"=w545) -> ("task out"=w546:refnum<k21>)  [unwired: 11 in, 2 out]
                    n125 = call <vilib>:"DAQmx Stop Task.vi"("task/channels in"=w546) -> ()  [unwired: 13 in, 2 out]
                  }
                }
              }
            }
            n126 = local read "H0"() -> (w381:dbl)
            n127 = call <vilib>:"Space Constant.vi"() -> ("String"=w366:string)
            n128 = call <vilib>:"Space Constant.vi"() -> ("String"=w361:string)
            n129 = Number To Fractional String(number=w357, precision (6)=i16 0) -> (F-format string=w367:string)  [unwired: 2 in]
            n130 = Number To Fractional String(number=w357, precision (6)=i16 0) -> (F-format string=w362:string)  [unwired: 2 in]
            n131 = call <vilib>:"Space Constant.vi"() -> ("String"=w422:string)
            n132 = call <vilib>:"Space Constant.vi"() -> ("String"=w442:string)
            n133 = call <vilib>:"Space Constant.vi"() -> ("String"=w409:string)
            n134 = call <vilib>:"Space Constant.vi"() -> ("String"=w433:string)
            n135 = call <vilib>:"Space Constant.vi"() -> ("String"=w399:string)
            n136 = Number To Fractional String(number=w357, precision (6)=i16 0) -> (F-format string=w425:string)  [unwired: 2 in]
            n137 = Number To Fractional String(number=w357, precision (6)=i16 0) -> (F-format string=w445:string)  [unwired: 2 in]
            n138 = Number To Fractional String(number=w357, precision (6)=i16 0) -> (F-format string=w412:string)  [unwired: 2 in]
            n139 = Number To Fractional String(number=w357, precision (6)=i16 0) -> (F-format string=w436:string)  [unwired: 2 in]
            n140 = Number To Fractional String(number=w357, precision (6)=i16 0) -> (F-format string=w402:string)  [unwired: 2 in]
            n141 = Concatenate Strings("trial", w366, w367, w366, "wind_history" ("string")) -> (w358:string)
            n142 = Concatenate Strings("trial", w361, w362, w361, "light_history") -> (w359:string)
            n143 = String To Path(string=w358) -> (path=w377:path)
            n144 = String To Path(string=w359) -> (path=w373:path)
            n145 = Concatenate Strings("trial", w422, w425, w422, "x_data") -> (w427:string)
            n146 = Concatenate Strings("trial", w442, w445, w442, "heading_data") -> (w447:string)
            n147 = Concatenate Strings("trial", w409, w412, w409, "LWBA_data") -> (w414:string)
            n148 = Concatenate Strings("trial", w433, w436, w433, "unfiltered deltaWBA") -> (w438:string)
            n149 = Concatenate Strings("trial", w399, w402, w399, "RWBA_data") -> (w404:string)
            n150 = Build Path(base path=w356, name or relative path=w377) -> (appended path=w374:path)
            n151 = Build Path(base path=w356, name or relative path=w373) -> (appended path=w371:path)
            n152 = String To Path(string=w427) -> (path=w428:path)
            n153 = Divide(x=w381, y=0.36) -> (x/y=w389:dbl)
            n154 = String To Path(string=w447) -> (path=w448:path)
            n155 = String To Path(string=w414) -> (path=w415:path)
            n156 = String To Path(string=w438) -> (path=w439:path)
            n157 = String To Path(string=w404) -> (path=w405:path)
            n158 = To Long Integer(number=w389) -> (32bit integer=w382:i32)
            n159 = Greater Than 0?(x=w382) -> (x > 0?=w388:bool)
            n160 = Not Equal To 0?(x=w382) -> (x != 0?=w383:bool)
            n161 = Build Path(base path=w356, name or relative path=w428) -> (appended path=w421:path)
            n162 = Build Path(base path=w356, name or relative path=w448) -> (appended path=w441:path)
            n163 = Build Path(base path=w356, name or relative path=w415) -> (appended path=w408:path)
            n164 = Build Path(base path=w356, name or relative path=w439) -> (appended path=w432:path)
            n165 = Build Path(base path=w356, name or relative path=w405) -> (appended path=w398:path)
            n166 = To Double Precision Float(number=w382) -> (double precision float=w385:dbl)
            n167 = Absolute Value(x=w382) -> (abs(x)=w387:i32)
            n168 = Multiply(x=0.36, y=w385) -> (x*y=w394:dbl)
            n169 = Open/Create/Replace File(file path (use dialog)=w374, operation (0:open)=T4."create", access (0:read/write)=enum16{"read/write", "read-only", "write-only"}."write-only") -> (refnum out=w355:refnum<file>)  [unwired: 3 in, 2 out]
            n170 = To Double Precision Float(number=w387) -> (double precision float=w386:dbl)
            n171 = case shown="True" w383 {
              tunnel: w388 -> [_ w454]
              tunnel: w386 -> [_ w453]
              frame False {
              }
              frame True {
                n172 = case shown="True" w454 {
                  tunnel: w453 -> [w455 w498]
                  frame True {
                    n173 = local read "Step Rate (Hz)"() -> (w458:dbl)
                    n174 = Reciprocal(x=w458) -> (1/x=w459:dbl)
                    n175 = node-c288(w459) -> (w461:T9)  [unwired: 3 in]
                    n176 = call-poly <vilib>:"DAQmx Create Virtual Channel.vi"("lines"=tag "Dev1/port0/line3") -> ("task out"=w457:refnum<k21>)  [unwired: 13 in, 1 out]
                    n177 = call-poly <vilib>:"DAQmx Create Virtual Channel.vi"("lines"=tag "Dev1/port0/line2") -> ("task out"=w456:refnum<k21>)  [unwired: 13 in, 1 out]
                    n178 = timed-loop {
                      timing: w461 -> [_]
                      timing-out: [_] -> w460
                      shift-right: [w474] -> _
                      shift-left: w457 -> [w472]
                      shift-right: [w473] -> _
                      shift-left: w456 -> [w471]
                      tunnel: w455 -> [w468]
                      i -> [w467]
                      stop <- w466 stop-if-true
                      n179 = node-c288() -> ()  [unwired: 1 in, 1 out]
                      n180 = flat-sequence {
                        tunnel: [w481] -> w476
                        tunnel: [w479] -> w475
                        tunnel: w472 -> [w478]
                        tunnel: w471 -> [w477]
                        tunnel: [w490] -> w474
                        tunnel: [w486] -> w473
                        tunnel: w476 -> [w489]
                        tunnel: w475 -> [w490]
                        frame #0 {
                          n181 = call-poly <vilib>:"DAQmx Write.vi"("task/channels in"=w478, "data"=FALSE) -> ("task out"=w480:refnum<k21>)  [unwired: 11 in, 2 out]
                          n182 = call-poly <vilib>:"DAQmx Write.vi"("task/channels in"=w477, "data"=TRUE) -> ("task out"=w482:refnum<k21>)  [unwired: 11 in, 2 out]
                          n183 = call <vilib>:"DAQmx Stop Task.vi"("task/channels in"=w480) -> ("task out"=w479:refnum<k21>)  [unwired: 13 in, 1 out]
                          n184 = call <vilib>:"DAQmx Stop Task.vi"("task/channels in"=w482) -> ("task out"=w481:refnum<k21>)  [unwired: 13 in, 1 out]
                        }
                        frame #1 {
                          n185 = call <vilib>:"DAQmx Start Task.vi"("task/channels in"=w489) -> ("task out"=w488:refnum<k21>)  [unwired: 13 in, 1 out]
                          n186 = call-poly <vilib>:"DAQmx Write.vi"("task/channels in"=w488, "data"=FALSE) -> ("task out"=w487:refnum<k21>)  [unwired: 11 in, 2 out]
                          n187 = call <vilib>:"DAQmx Stop Task.vi"("task/channels in"=w487) -> ("task out"=w486:refnum<k21>)  [unwired: 13 in, 1 out]
                        }
                      }
                      n188 = To Double Precision Float(number=w467) -> (double precision float=w469:dbl)
                      n189 = Increment(x=w469) -> (x+1=w470:dbl)
                      n190 = local read "Motor Error"() -> (w464:bool)
                      n191 = Equal?(x=w468, y=w470) -> (x = y?=w465:bool)
                      n192 = Or(x=w464, y=w465) -> (x .or. y?=w466:bool)
                      n193 = node-c288() -> ()  [unwired: 1 in, 1 out]
                    }
                    n194 = node-c288(w460) -> ()  [unwired: 1 out]
                  }
                  frame False {
                    n195 = local read "Step Rate (Hz)"() -> (w501:dbl)
                    n196 = Reciprocal(x=w501) -> (1/x=w502:dbl)
                    n197 = node-c288(w502) -> (w504:T9)  [unwired: 3 in]
                    n198 = call-poly <vilib>:"DAQmx Create Virtual Channel.vi"("lines"=tag "Dev1/port0/line3") -> ("task out"=w500:refnum<k21>)  [unwired: 13 in, 1 out]
                    n199 = call-poly <vilib>:"DAQmx Create Virtual Channel.vi"("lines"=tag "Dev1/port0/line2") -> ("task out"=w499:refnum<k21>)  [unwired: 13 in, 1 out]
                    n200 = timed-loop {
                      timing: w504 -> [_]
                      timing-out: [_] -> w503
                      shift-right: [w516] -> _
                      shift-left: w500 -> [w517]
                      shift-right: [w514] -> _
                      shift-left: w499 -> [w515]
                      tunnel: w498 -> [w510]
                      i -> [w509]
                      stop <- w508 stop-if-true
                      n201 = node-c288() -> ()  [unwired: 1 in, 1 out]
                      n202 = flat-sequence {
                        tunnel: [w524] -> w519
                        tunnel: [w522] -> w518
                        tunnel: w515 -> [w521]
                        tunnel: w517 -> [w520]
                        tunnel: [w533] -> w514
                        tunnel: [w529] -> w516
                        tunnel: w519 -> [w532]
                        tunnel: w518 -> [w533]
                        frame #0 {
                          n203 = call-poly <vilib>:"DAQmx Write.vi"("task/channels in"=w521, "data"=FALSE) -> ("task out"=w523:refnum<k21>)  [unwired: 11 in, 2 out]
                          n204 = call-poly <vilib>:"DAQmx Write.vi"("task/channels in"=w520, "data"=TRUE) -> ("task out"=w525:refnum<k21>)  [unwired: 11 in, 2 out]
                          n205 = call <vilib>:"DAQmx Stop Task.vi"("task/channels in"=w523) -> ("task out"=w522:refnum<k21>)  [unwired: 13 in, 1 out]
                          n206 = call <vilib>:"DAQmx Stop Task.vi"("task/channels in"=w525) -> ("task out"=w524:refnum<k21>)  [unwired: 13 in, 1 out]
                        }
                        frame #1 {
                          n207 = call <vilib>:"DAQmx Start Task.vi"("task/channels in"=w532) -> ("task out"=w531:refnum<k21>)  [unwired: 13 in, 1 out]
                          n208 = call-poly <vilib>:"DAQmx Write.vi"("task/channels in"=w531, "data"=FALSE) -> ("task out"=w530:refnum<k21>)  [unwired: 11 in, 2 out]
                          n209 = call <vilib>:"DAQmx Stop Task.vi"("task/channels in"=w530) -> ("task out"=w529:refnum<k21>)  [unwired: 13 in, 1 out]
                        }
                      }
                      n210 = To Double Precision Float(number=w509) -> (double precision float=w512:dbl)
                      n211 = Increment(x=w512) -> (x+1=w513:dbl)
                      n212 = Equal?(x=w510, y=w513) -> (x = y?=w511:bool)
                      n213 = local read "Motor Error"() -> (w507:bool)
                      n214 = Or(x=w507, y=w511) -> (x .or. y?=w508:bool)
                      n215 = node-c288() -> ()  [unwired: 1 in, 1 out]
                    }
                    n216 = node-c288(w503) -> ()  [unwired: 1 out]
                  }
                }
              }
            }
            n217 = Open/Create/Replace File(file path (use dialog)=w371, operation (0:open)=T4."create", access (0:read/write)=enum16{"read/write", "read-only", "write-only"}."write-only") -> (refnum out=w354:refnum<file>)  [unwired: 3 in, 2 out]
            n218 = Open/Create/Replace File(file path (use dialog)=w421, operation (0:open)=T4."create", access (0:read/write)=enum16{"read/write", "read-only", "write-only"}."write-only") -> (refnum out=w419:refnum<file>)  [unwired: 3 in, 2 out]
            n219 = Open/Create/Replace File(file path (use dialog)=w441, operation (0:open)=T4."create", access (0:read/write)=enum16{"read/write", "read-only", "write-only"}."write-only") -> (refnum out=w418:refnum<file>)  [unwired: 3 in, 2 out]
            n220 = Open/Create/Replace File(file path (use dialog)=w408, operation (0:open)=T4."create", access (0:read/write)=enum16{"read/write", "read-only", "write-only"}."write-only") -> (refnum out=w396:refnum<file>)  [unwired: 3 in, 2 out]
            n221 = Open/Create/Replace File(file path (use dialog)=w432, operation (0:open)=T4."create", access (0:read/write)=enum16{"read/write", "read-only", "write-only"}."write-only") -> (refnum out=w417:refnum<file>)  [unwired: 3 in, 2 out]
            n222 = Open/Create/Replace File(file path (use dialog)=w398, operation (0:open)=T4."create", access (0:read/write)=enum16{"read/write", "read-only", "write-only"}."write-only") -> (refnum out=w395:refnum<file>)  [unwired: 3 in, 2 out]
            n223 = local write "Heading (deg)"(w394) -> ()
            n224 = local write "H"(w394) -> ()
          }
          frame #3 {
            n225 = call-poly <vilib>:"DAQmx Create Virtual Channel.vi"("lines"=tag "Dev1/port0/line3") -> ("task out"=w569:refnum<k21>)  [unwired: 13 in, 1 out]
            n226 = call-poly <vilib>:"DAQmx Create Virtual Channel.vi"("lines"=tag "Dev1/port0/line2") -> ("task out"=w570:refnum<k21>)  [unwired: 13 in, 1 out]
            n227 = call-poly <vilib>:"DAQmx Create Virtual Channel.vi"("lines"=tag "Dev1/port0/line6") -> ("task out"=w562:refnum<k21>)  [unwired: 13 in, 1 out]
            n228 = call-poly <vilib>:"DAQmx Create Virtual Channel.vi"("physical channels"=tag "Dev1/ao0") -> ("task out"=w559:refnum<k21>)  [unwired: 13 in, 1 out]
            n229 = Reciprocal(x="Data Rate (Hz)") -> (1/x=w553:dbl)
            n230 = call-poly <vilib>:"DAQmx Create Virtual Channel.vi"("lines"=tag "Dev1/port0/line1") -> ("task out"=w565:refnum<k21>)  [unwired: 13 in, 1 out]
            n231 = node-c288(w553) -> (w588:T9)  [unwired: 3 in]
            n232 = timed-loop {
              timing: w588 -> [_]
              timing-out: [_] -> w587
              tunnel: w585 -> [w681]
              tunnel: w584 -> [w682]
              tunnel: w583 -> [w680]
              shift-right: [w664] -> w579
              shift-left: w570 -> [w666]
              shift-right: [w665] -> w580
              shift-left: w569 -> [w667]
              tunnel: w582 -> [w679]
              tunnel: [w678] -> w581
              shift-right: [w676] -> _
              shift-left: w564 -> [w677]
              tunnel: w578 -> [w675]
              tunnel: [w674] -> w577
              tunnel: [w673] -> w576
              tunnel: w575 -> [w672]
              tunnel: w574 -> [w671]
              tunnel: w573 -> [w670]
              tunnel: [w669] -> w572
              tunnel: [w668] -> w571
              shift-right: [w660] -> _
              shift-left: w565 -> [w663]
              shift-right: [w604] -> _
              shift-left: _ -> [w618]
              shift-right: [w613] -> w561
              shift-left: w562 -> [w616]
              shift-right: [w605] -> w558
              shift-left: w559 -> [w606]
              tunnel: w555 -> [w603]
              tunnel: w554 -> [w602]
              tunnel: w552 -> [w595]
              tunnel: w551 -> [w594]
              tunnel: [w591] -> w550
              tunnel: [w590] -> w549
              i -> [w596]
              stop <- w657 stop-if-true
              w646 = T15 {"Search Direction"=0, "Edge Options"={"Edge Polarity"=0, "Kernel Size"=3, "Width"=3, "Minimum Edge Strength"=2.0, "Interpolation Type"=enum."Bilinear Fixed", "Data Processing Method"=enum."Average"}, "Show Search Area"=TRUE, "Show Search Lines"=TRUE, "Show Edges Found"=TRUE, "Show Result"=TRUE, "Search Area Color"=65280, "Search Lines Color"=255, "Edge Locations Color"=16776960, "Result Color"=16711680, "Overlay Group Name"=""} ("Options")
              n233 = node-c288() -> ()  [unwired: 1 in, 1 out]
              n234 = To Double Precision Float(number=w596) -> (double precision float=w622:dbl)
              n235 = local read "Data Rate (Hz)"() -> (w589:dbl)
              n236 = local read "Data Rate (Hz)"() -> (w637:dbl)
              n237 = Increment(x=w622) -> (x+1=w633:dbl)
              n238 = call <vilib>:"DAQmx Start Task.vi"("task/channels in"=w616) -> ("task out"=w615:refnum<k21>)  [unwired: 13 in, 1 out]
              n239 = Multiply(x=w589, y="Stimulus Duration (s)") -> (x*y=w597:dbl)
              n240 = Less?(x=w596, y=w597) -> (x < y?=w599:bool)
              n241 = case shown="True" w599 {
                tunnel: w603 -> [_ w689]
                tunnel: w602 -> [_ w688]
                tunnel: w596 -> [_ w685]
                tunnel: [w684 w687] -> w601
                tunnel: [w683 w686] -> w600
                frame False {
                  w683 = TRUE ("Light")
                  w684 = FALSE ("Wind")
                  n242 = local write "Wind"(w684) -> ()
                  n243 = local write "Light"(w683) -> ()
                }
                frame True {
                  n244 = Index Array(array=w689, index=w685) -> (element=w691:dbl)
                  n245 = Index Array(array=w688, index=w685) -> (element=w690:dbl)
                  n246 = Equal?(x=1.0, y=w691) -> (x = y?=w686:bool)
                  n247 = Equal?(x=1.0, y=w690) -> (x = y?=w687:bool)
                  n248 = local write "Light"(w686) -> ()
                  n249 = local write "Wind"(w687) -> ()
                }
              }
              n250 = Boolean To (0,1)(Boolean=w600) -> (0, 1=w593:i16)
              "Light History" <- w593
              n251 = call <vilib>:"DAQmx Start Task.vi"("task/channels in"=w663) -> ("task out"=w662:refnum<k21>)  [unwired: 13 in, 1 out]
              n252 = Boolean To (0,1)(Boolean=w601) -> (0, 1=w592:i16)
              "Wind History" <- w592
              n253 = Divide(x=w633, y=w637) -> (x/y=w636:dbl)
              n254 = call-poly <vilib>:"DAQmx Write.vi"("task/channels in"=w615, "data"=w601) -> ("task out"=w614:refnum<k21>)  [unwired: 11 in, 2 out]
              n255 = call "IMAQ Create"("Image Name"="flyim") -> ("New Image"=w656:T3)  [unwired: 3 in, 2 out]
              n256 = Greater?(x=w636, y="Trial Duration (s)") -> (0:→"Trial End":bool)
              n257 = call <vilib>:"DAQmx Stop Task.vi"("task/channels in"=w614) -> ("task out"=w613:refnum<k21>)  [unwired: 13 in, 1 out]
              n258 = call-poly <vilib>:"DAQmx Read.vi"("task/channels in"=w662) -> ("task out"=w661:refnum<k21>, "data"=→"Motor Error":bool)  [unwired: 12 in, 1 out]
              n259 = call <vilib>:"IMAQdx Grab.vi"("Wait for Next Buffer? (Yes)"=FALSE, "Image In"=w656, "Session In"=w682) -> ("Image Out"=w647:T3)  [unwired: 1 in, 7 out]
              n260 = call "IMAQ Threshold"("Keep/Replace Value (Replace)"=FALSE, "Range"="Image Threshold", "Image Src"=w647) -> ("Image Dst Out"=w652:T3)  [unwired: 7 in, 1 out]
              n261 = call <vilib>:"DAQmx Stop Task.vi"("task/channels in"=w661) -> ("task out"=w660:refnum<k21>)  [unwired: 13 in, 1 out]
              n262 = call "IMAQ Find Edge"("Line Fit Options"="L options", "Options"=w646, "ROI Descriptor"=w681, "Image"=w652) -> ("Straight Edges"=w649:T16, "Image Out"=w651:T3)  [unwired: 4 in, 2 out]
              n263 = case shown="True" w600 {
                tunnel: w606 -> [w698 w701]
                tunnel: [w696 w700] -> w605
                frame False {
                  n264 = call <vilib>:"DAQmx Start Task.vi"("task/channels in"=w698) -> ("task out"=w697:refnum<k21>)  [unwired: 13 in, 1 out]
                  n265 = call-poly <vilib>:"DAQmx Write.vi"("task/channels in"=w697, "data"=0.0) -> ("task out"=w695:refnum<k21>)  [unwired: 11 in, 2 out]
                  n266 = call <vilib>:"DAQmx Stop Task.vi"("task/channels in"=w695) -> ("task out"=w696:refnum<k21>)  [unwired: 13 in, 1 out]
                }
                frame True {
                  n267 = call <vilib>:"DAQmx Start Task.vi"("task/channels in"=w701) -> ("task out"=w703:refnum<k21>)  [unwired: 13 in, 1 out]
                  n268 = local read "Light Intensity (V)"() -> (w699:dbl)
                  n269 = call-poly <vilib>:"DAQmx Write.vi"("task/channels in"=w703, "data"=w699) -> ("task out"=w702:refnum<k21>)  [unwired: 11 in, 2 out]
                  n270 = call <vilib>:"DAQmx Stop Task.vi"("task/channels in"=w702) -> ("task out"=w700:refnum<k21>)  [unwired: 13 in, 1 out]
                }
              }
              n271 = Write to Binary File(file (use dialog)=w595, data=w592) -> (refnum out=w591:refnum<file>)  [unwired: 4 in, 2 out]
              n272 = Write to Binary File(file (use dialog)=w594, data=w593) -> (refnum out=w590:refnum<file>)  [unwired: 4 in, 2 out]
              n273 = call "IMAQ Find Edge"("Line Fit Options"="R options", "Options"=w646, "ROI Descriptor"=w680, "Image"=w651) -> ("Straight Edges"=w648:T16, "Image Out"=→"Image":T3)  [unwired: 4 in, 2 out]
              n274 = Array To Cluster(array=w648) -> (cluster=w639:T17)
              n275 = Array To Cluster(array=w649) -> (cluster=w638:T17)
              n276 = Unbundle By Name(w639) -> ("Straight Edges[0].Angle (Pixel)"=w644:dbl)
              n277 = Unbundle By Name(w638) -> ("Straight Edges[0].Angle (Pixel)"=w645:dbl)
              n278 = Absolute Value(x=w644) -> (abs(x)=w623:dbl)
              "L WBA" <- w623
              n279 = Absolute Value(x=w645) -> (abs(x)=w624:dbl)
              "R WBA" <- w624
              n280 = Write to Binary File(file (use dialog)=w670, data=w624) -> (refnum out=w669:refnum<file>)  [unwired: 4 in, 2 out]
              n281 = Write to Binary File(file (use dialog)=w671, data=w623) -> (refnum out=w668:refnum<file>)  [unwired: 4 in, 2 out]
              n282 = Subtract(x=w623, y=w624) -> (x-y=w642:dbl)
              "L-R WBA" <- w642
              n283 = case shown="True" "Reversed Tether?" {
                tunnel: w642 -> [w706 w708]
                tunnel: [w705 w707] -> w641
                tunnel: "L-R WBA Offset (deg)" -> [w704 w709]
                frame False {
                  n284 = Add ("Add.vi")(x=w706, y=w704) -> (x+y=w705:dbl)
                }
                frame True {
                  n285 = Subtract(x=w708, y=w709) -> (x-y=w707:dbl)
                }
              }
              n286 = Multiply(x=w641, y="deltaWBA Gain (g, unitless)") -> (x*y=w643:dbl)
              n287 = case shown="True" "Reversed Tether?" {
                tunnel: w643 -> [w711 w712]
                tunnel: [w710 w712] -> w610
                frame False {
                  n288 = Negate(x=w711) -> (-x=w710:dbl)
                }
                frame True {
                }
              }
              "Scaled deltaWBA (deg)" <- w610
              "deltaWBA" <- w610
              n289 = Greater Or Equal To 0?(x=w610) -> (x >= 0?=w611:bool)
              n290 = case shown="True" w611 {
                tunnel: [w723 w740] -> w604
                tunnel: "Max steps/sample" -> [w722 w736]
                tunnel: w610 -> [w716 w735]
                frame False {
                  n291 = Absolute Value(x=w716) -> (abs(x)=w717:dbl)
                  n292 = Quotient & Remainder(x=w717, y=0.36) -> (x-y*floor(x/y)=w715:dbl, floor(x/y)=w718:dbl)
                  n293 = Greater?(x=w715, y=0.18) -> (0:w719:bool)
                  n294 = Negate(x=w722) -> (-x=w724:dbl)
                  n295 = case shown="True" w719 {
                    tunnel: w718 -> [w726 w729]
                    tunnel: [w726 w727] -> w714
                    frame False {
                    }
                    frame True {
                      n296 = Add(x=w729, y=1.0) -> (x+y=w727:dbl)
                    }
                  }
                  n297 = Negate(x=w714) -> (-x=w713:dbl)
                  n298 = Less?(x=w713, y=w724) -> (x < y?=w725:bool)
                  n299 = case shown="False" w725 {
                    tunnel: w724 -> [_ w731]
                    tunnel: [w730 w731] -> w723
                    tunnel: w713 -> [w730 _]
                    frame False {
                    }
                    frame True {
                    }
                  }
                }
                frame True {
                  n300 = Quotient & Remainder(x=w735, y=0.36) -> (x-y*floor(x/y)=w733:dbl, floor(x/y)=w738:dbl)
                  n301 = Greater?(x=w733, y=0.18) -> (0:w734:bool)
                  n302 = case shown="True" w734 {
                    tunnel: w738 -> [w742 w745]
                    tunnel: [w742 w743] -> w739
                    frame False {
                    }
                    frame True {
                      n303 = Add(x=w745, y=1.0) -> (x+y=w743:dbl)
                    }
                  }
                  n304 = Greater?(x=w739, y=w736) -> (0:w741:bool)
                  n305 = case shown="False" w741 {
                    tunnel: w736 -> [_ w747]
                    tunnel: [w746 w747] -> w740
                    tunnel: w739 -> [w746 _]
                    frame False {
                    }
                    frame True {
                    }
                  }
                }
              }
              "X (steps/sample)" <- w604
              n306 = Multiply(x=0.36 ("y"), y=w604) -> (x*y=w625:dbl)
              n307 = Add ("Add.vi")(x=w625, y=w677) -> (x+y=w629:dbl)
              n308 = Add(x=w629, y=180.0 ("x")) -> (x+y=w630:dbl)
              n309 = Quotient & Remainder(x=w630, y=360.0) -> (x-y*floor(x/y)=w631:dbl)  [unwired: 1 out]
              n310 = Subtract(x=w631, y=180.0) -> (x-y=w676:dbl)
              "H" <- w676
              "Heading (deg)" <- w676
              n311 = Write to Binary File(file (use dialog)=w675, data=w676) -> (refnum out=w674:refnum<file>)  [unwired: 4 in, 2 out]
              n312 = Write to Binary File(file (use dialog)=w672, data=w610) -> (refnum out=w678:refnum<file>)  [unwired: 4 in, 2 out]
              n313 = Write to Binary File(file (use dialog)=w679, data=w604) -> (refnum out=w673:refnum<file>)  [unwired: 4 in, 2 out]
              n314 = Not Equal To 0?(x=w618) -> (x != 0?=w619:bool)
              n315 = case shown="True" w619 {
                tunnel: w667 -> [w749 w756]
                tunnel: w666 -> [w748 w755]
                tunnel: w618 -> [_ w754]
                tunnel: [w748 w753] -> w664
                tunnel: [w749 w752] -> w665
                frame False {
                }
                frame True {
                  n316 = Reciprocal(x="Step Rate (Hz)") -> (1/x=w750:dbl)
                  n317 = node-c288(w750) -> (w758:T9)  [unwired: 3 in]
                  n318 = timed-loop {
                    timing: w758 -> [_]
                    timing-out: [_] -> w757
                    tunnel: w754 -> [w772]
                    shift-right: [w765] -> w752
                    shift-left: w756 -> [w769]
                    shift-right: [w764] -> w753
                    shift-left: w755 -> [w767]
                    i -> [w763]
                    stop <- w761 stop-if-true
                    n319 = node-c288() -> ()  [unwired: 1 in, 1 out]
                    n320 = To Double Precision Float(number=w763) -> (double precision float=w762:dbl)
                    n321 = Absolute Value(x=w772) -> (abs(x)=w771:dbl)
                    n322 = call <vilib>:"DAQmx Start Task.vi"("task/channels in"=w769) -> ("task out"=w768:refnum<k21>)  [unwired: 13 in, 1 out]
                    n323 = call <vilib>:"DAQmx Start Task.vi"("task/channels in"=w767) -> ("task out"=w766:refnum<k21>)  [unwired: 13 in, 1 out]
                    n324 = Increment(x=w762) -> (x+1=w770:dbl)
                    n325 = Greater Than 0?(x=w772) -> (x > 0?=w773:bool)
                    n326 = Equal?(x=w771, y=w770) -> (x = y?=w760:bool)
                    n327 = case shown="False" w773 {
                      tunnel: [w776 w796] -> w765
                      tunnel: [w777 w797] -> w764
                      tunnel: w766 -> [w779 w799]
                      tunnel: w768 -> [w778 w798]
                      frame True {
                        n328 = flat-sequence {
                          tunnel: w779 -> [w787]
                          tunnel: w778 -> [w786]
                          tunnel: [w782] -> w775
                          tunnel: [w780] -> w774
                          tunnel: [w793] -> w776
                          tunnel: [w789] -> w777
                          tunnel: w775 -> [w792]
                          tunnel: w774 -> [w793]
                          frame #0 {
                            n329 = call-poly <vilib>:"DAQmx Write.vi"("task/channels in"=w786, "data"=FALSE) -> ("task out"=w781:refnum<k21>)  [unwired: 11 in, 2 out]
                            n330 = call-poly <vilib>:"DAQmx Write.vi"("task/channels in"=w787, "data"=TRUE) -> ("task out"=w783:refnum<k21>)  [unwired: 11 in, 2 out]
                            n331 = call <vilib>:"DAQmx Stop Task.vi"("task/channels in"=w781) -> ("task out"=w780:refnum<k21>)  [unwired: 13 in, 1 out]
                            n332 = call <vilib>:"DAQmx Stop Task.vi"("task/channels in"=w783) -> ("task out"=w782:refnum<k21>)  [unwired: 13 in, 1 out]
                          }
                          frame #1 {
                            n333 = call <vilib>:"DAQmx Start Task.vi"("task/channels in"=w792) -> ("task out"=w791:refnum<k21>)  [unwired: 13 in, 1 out]
                            n334 = call-poly <vilib>:"DAQmx Write.vi"("task/channels in"=w791, "data"=FALSE) -> ("task out"=w790:refnum<k21>)  [unwired: 11 in, 2 out]
                            n335 = call <vilib>:"DAQmx Stop Task.vi"("task/channels in"=w790) -> ("task out"=w789:refnum<k21>)  [unwired: 13 in, 1 out]
                          }
                        }
                      }
                      frame False {
                        n336 = flat-sequence {
                          tunnel: w799 -> [w807]
                          tunnel: w798 -> [w806]
                          tunnel: [w802] -> w795
                          tunnel: [w800] -> w794
                          tunnel: [w809] -> w796
                          tunnel: [w808] -> w797
                          tunnel: w795 -> [w808]
                          tunnel: w794 -> [w810]
                          frame #0 {
                            n337 = call-poly <vilib>:"DAQmx Write.vi"("task/channels in"=w806, "data"=TRUE) -> ("task out"=w801:refnum<k21>)  [unwired: 11 in, 2 out]
                            n338 = call-poly <vilib>:"DAQmx Write.vi"("task/channels in"=w807, "data"=FALSE) -> ("task out"=w803:refnum<k21>)  [unwired: 11 in, 2 out]
                            n339 = call <vilib>:"DAQmx Stop Task.vi"("task/channels in"=w801) -> ("task out"=w800:refnum<k21>)  [unwired: 13 in, 1 out]
                            n340 = call <vilib>:"DAQmx Stop Task.vi"("task/channels in"=w803) -> ("task out"=w802:refnum<k21>)  [unwired: 13 in, 1 out]
                          }
                          frame #1 {
                            n341 = call <vilib>:"DAQmx Start Task.vi"("task/channels in"=w810) -> ("task out"=w813:refnum<k21>)  [unwired: 13 in, 1 out]
                            n342 = call-poly <vilib>:"DAQmx Write.vi"("task/channels in"=w813, "data"=FALSE) -> ("task out"=w812:refnum<k21>)  [unwired: 11 in, 2 out]
                            n343 = call <vilib>:"DAQmx Stop Task.vi"("task/channels in"=w812) -> ("task out"=w809:refnum<k21>)  [unwired: 13 in, 1 out]
                          }
                        }
                      }
                    }
                    n344 = local read "Motor Error"() -> (w759:bool)
                    n345 = Or(x=w760, y=w759) -> (x .or. y?=w761:bool)
                    n346 = node-c288() -> ()  [unwired: 1 in, 1 out]
                  }
                  n347 = node-c288(w757) -> ()  [unwired: 1 out]
                }
              }
              n348 = local read "Motor Error"() -> (w658:bool)
              n349 = local read "Trial End"() -> (w659:bool)
              n350 = Or(x=w659, y=w658) -> (x .or. y?=w657:bool)
              n351 = node-c288() -> ()  [unwired: 1 in, 1 out]
            }
            n352 = node-c288(w587) -> ()  [unwired: 1 out]
          }
          frame #4 {
            n353 = local read "H"() -> (w838:dbl)
            n354 = Close File(refnum=w829) -> ()  [unwired: 1 in, 2 out]
            n355 = Close File(refnum=w828) -> ()  [unwired: 1 in, 2 out]
            n356 = Absolute Value(x=w838) -> (abs(x)=w832:dbl)
            n357 = Close File(refnum=w848) -> ()  [unwired: 1 in, 2 out]
            n358 = Close File(refnum=w847) -> ()  [unwired: 1 in, 2 out]
            n359 = Close File(refnum=w846) -> ()  [unwired: 1 in, 2 out]
            n360 = Close File(refnum=w845) -> ()  [unwired: 1 in, 2 out]
            n361 = Close File(refnum=w849) -> ()  [unwired: 1 in, 2 out]
            n362 = Greater Than 0?(x=w838) -> (x > 0?=w844:bool)
            n363 = To Long Integer(number=w832) -> (32bit integer=w831:i32)
            n364 = Not Equal To 0?(x=w831) -> (x != 0?=w843:bool)
            n365 = case shown="True" w843 {
              tunnel: w851 -> [_ w855]
              tunnel: w850 -> [_ w854]
              tunnel: w844 -> [_ w853]
              tunnel: w838 -> [_ w852]
              frame False {
              }
              frame True {
                n366 = case shown="False" w853 {
                  tunnel: w855 -> [w866 w917]
                  tunnel: w854 -> [w865 w916]
                  tunnel: w852 -> [w863 w914]
                  frame True {
                    n367 = local read "X (steps/sample)"() -> (w857:dbl)
                    n368 = Divide(x=w863, y=0.36) -> (x/y=w859:dbl)
                    n369 = Add(x=1.0, y=w857) -> (x+y=w858:dbl)
                    n370 = Subtract(x=w859, y=w858) -> (x-y=w861:dbl)
                    n371 = local read "Step Rate (Hz)"() -> (w864:dbl)
                    n372 = Reciprocal(x=w864) -> (1/x=w867:dbl)
                    n373 = node-c288(w867) -> (w869:T9)  [unwired: 3 in]
                    n374 = Absolute Value(x=w861) -> (abs(x)=w860:dbl)
                    n375 = timed-loop {
                      timing: w869 -> [_]
                      timing-out: [_] -> w868
                      shift-right: [w881] -> _
                      shift-left: w865 -> [w879]
                      shift-right: [w882] -> _
                      shift-left: w866 -> [w880]
                      tunnel: w860 -> [w873]
                      i -> [w871]
                      stop <- w876 stop-if-true
                      n376 = node-c288() -> ()  [unwired: 1 in, 1 out]
                      n377 = To Long Integer(number=w871) -> (32bit integer=w870:i32)
                      n378 = To Long Integer(number=w873) -> (32bit integer=w872:i32)
                      n379 = flat-sequence {
                        tunnel: w880 -> [w889]
                        tunnel: w879 -> [w887]
                        tunnel: [w892] -> w878
                        tunnel: [w890] -> w877
                        tunnel: [w899] -> w881
                        tunnel: [w894] -> w882
                        tunnel: w878 -> [w897]
                        tunnel: w877 -> [w899]
                        frame #0 {
                          n380 = call <vilib>:"DAQmx Start Task.vi"("task/channels in"=w889) -> ("task out"=w888:refnum<k21>)  [unwired: 13 in, 1 out]
                          n381 = call <vilib>:"DAQmx Start Task.vi"("task/channels in"=w887) -> ("task out"=w886:refnum<k21>)  [unwired: 13 in, 1 out]
                          n382 = call-poly <vilib>:"DAQmx Write.vi"("task/channels in"=w888, "data"=TRUE) -> ("task out"=w893:refnum<k21>)  [unwired: 11 in, 2 out]
                          n383 = call-poly <vilib>:"DAQmx Write.vi"("task/channels in"=w886, "data"=FALSE) -> ("task out"=w891:refnum<k21>)  [unwired: 11 in, 2 out]
                          n384 = call <vilib>:"DAQmx Stop Task.vi"("task/channels in"=w893) -> ("task out"=w892:refnum<k21>)  [unwired: 13 in, 1 out]
                          n385 = call <vilib>:"DAQmx Stop Task.vi"("task/channels in"=w891) -> ("task out"=w890:refnum<k21>)  [unwired: 13 in, 1 out]
                        }
                        frame #1 {
                          n386 = call <vilib>:"DAQmx Start Task.vi"("task/channels in"=w897) -> ("task out"=w896:refnum<k21>)  [unwired: 13 in, 1 out]
                          n387 = call-poly <vilib>:"DAQmx Write.vi"("task/channels in"=w896, "data"=FALSE) -> ("task out"=w895:refnum<k21>)  [unwired: 11 in, 2 out]
                          n388 = call <vilib>:"DAQmx Stop Task.vi"("task/channels in"=w895) -> ("task out"=w894:refnum<k21>)  [unwired: 13 in, 1 out]
                        }
                      }
                      n389 = Increment(x=w870) -> (x+1=w883:i32)
                      n390 = Equal?(x=w872, y=w883) -> (x = y?=w874:bool)
                      n391 = local read "Motor Error"() -> (w875:bool)
                      n392 = Or(x=w875, y=w874) -> (x .or. y?=w876:bool)
                      n393 = node-c288() -> ()  [unwired: 1 in, 1 out]
                    }
                    n394 = node-c288(w868) -> ()  [unwired: 1 out]
                  }
                  frame False {
                    n395 = local read "X (steps/sample)"() -> (w909:dbl)
                    n396 = Divide(x=w914, y=0.36) -> (x/y=w912:dbl)
                    n397 = Add(x=1.0, y=w909) -> (x+y=w907:dbl)
                    n398 = local read "Step Rate (Hz)"() -> (w915:dbl)
                    n399 = Reciprocal(x=w915) -> (1/x=w918:dbl)
                    n400 = node-c288(w918) -> (w920:T9)  [unwired: 3 in]
                    n401 = Subtract(x=w912, y=w907) -> (x-y=w911:dbl)
                    n402 = Absolute Value(x=w911) -> (abs(x)=w910:dbl)
                    n403 = timed-loop {
                      timing: w920 -> [_]
                      timing-out: [_] -> w919
                      shift-right: [w932] -> _
                      shift-left: w916 -> [w930]
                      shift-right: [w933] -> _
                      shift-left: w917 -> [w931]
                      tunnel: w910 -> [w922]
                      i -> [w924]
                      stop <- w927 stop-if-true
                      n404 = node-c288() -> ()  [unwired: 1 in, 1 out]
                      n405 = To Long Integer(number=w922) -> (32bit integer=w921:i32)
                      n406 = To Long Integer(number=w924) -> (32bit integer=w923:i32)
                      n407 = flat-sequence {
                        tunnel: w931 -> [w940]
                        tunnel: w930 -> [w938]
                        tunnel: [w943] -> w929
                        tunnel: [w941] -> w928
                        tunnel: [w946] -> w932
                        tunnel: [w945] -> w933
                        tunnel: w929 -> [w945]
                        tunnel: w928 -> [w947]
                        frame #0 {
                          n408 = call <vilib>:"DAQmx Start Task.vi"("task/channels in"=w940) -> ("task out"=w939:refnum<k21>)  [unwired: 13 in, 1 out]
                          n409 = call <vilib>:"DAQmx Start Task.vi"("task/channels in"=w938) -> ("task out"=w937:refnum<k21>)  [unwired: 13 in, 1 out]
                          n410 = call-poly <vilib>:"DAQmx Write.vi"("task/channels in"=w939, "data"=FALSE) -> ("task out"=w944:refnum<k21>)  [unwired: 11 in, 2 out]
                          n411 = call-poly <vilib>:"DAQmx Write.vi"("task/channels in"=w937, "data"=TRUE) -> ("task out"=w942:refnum<k21>)  [unwired: 11 in, 2 out]
                          n412 = call <vilib>:"DAQmx Stop Task.vi"("task/channels in"=w944) -> ("task out"=w943:refnum<k21>)  [unwired: 13 in, 1 out]
                          n413 = call <vilib>:"DAQmx Stop Task.vi"("task/channels in"=w942) -> ("task out"=w941:refnum<k21>)  [unwired: 13 in, 1 out]
                        }
                        frame #1 {
                          n414 = call <vilib>:"DAQmx Start Task.vi"("task/channels in"=w947) -> ("task out"=w949:refnum<k21>)  [unwired: 13 in, 1 out]
                          n415 = call-poly <vilib>:"DAQmx Write.vi"("task/channels in"=w949, "data"=FALSE) -> ("task out"=w948:refnum<k21>)  [unwired: 11 in, 2 out]
                          n416 = call <vilib>:"DAQmx Stop Task.vi"("task/channels in"=w948) -> ("task out"=w946:refnum<k21>)  [unwired: 13 in, 1 out]
                        }
                      }
                      n417 = Increment(x=w923) -> (x+1=w934:i32)
                      n418 = Equal?(x=w921, y=w934) -> (x = y?=w926:bool)
                      n419 = local read "Motor Error"() -> (w925:bool)
                      n420 = Or(x=w925, y=w926) -> (x .or. y?=w927:bool)
                      n421 = node-c288() -> ()  [unwired: 1 in, 1 out]
                    }
                    n422 = node-c288(w919) -> ()  [unwired: 1 out]
                  }
                }
              }
            }
            n423 = call <vilib>:"DAQmx Start Task.vi"("task/channels in"=w835) -> ("task out"=w837:refnum<k21>)  [unwired: 13 in, 1 out]
            n424 = call <vilib>:"DAQmx Start Task.vi"("task/channels in"=w841) -> ("task out"=w840:refnum<k21>)  [unwired: 13 in, 1 out]
            n425 = call-poly <vilib>:"DAQmx Write.vi"("task/channels in"=w837, "data"=0.0) -> ("task out"=w836:refnum<k21>)  [unwired: 11 in, 2 out]
            n426 = call-poly <vilib>:"DAQmx Write.vi"("task/channels in"=w840, "data"=FALSE) -> ("task out"=w839:refnum<k21>)  [unwired: 11 in, 2 out]
            n427 = call <vilib>:"DAQmx Stop Task.vi"("task/channels in"=w836) -> ()  [unwired: 13 in, 2 out]
            n428 = call <vilib>:"DAQmx Stop Task.vi"("task/channels in"=w839) -> ()  [unwired: 13 in, 2 out]
          }
          frame #5 {
            n429 = Unbundle(w973) -> ("y"=w967:i32, "y"=w966:i32, "y"=w965:i32, "y"=w964:i32, "y"=w961:i32, "y"=w960:i32)
            n430 = Greater?(x=w963, y=3.0) -> (0:w962:bool)
            n431 = case shown="False" w962 {
              tunnel: [w993 w1044] -> w972
              tunnel: [w992 w1043] -> w971
              tunnel: [w991 w1042] -> w970
              tunnel: [w990 w1041] -> w969
              tunnel: w967 -> [w989 w1040]
              tunnel: w966 -> [w988 w1039]
              tunnel: w965 -> [w987 w1038]
              tunnel: w964 -> [w986 w1037]
              tunnel: w963 -> [w979 w1030]
              tunnel: w961 -> [w983 w1034]
              tunnel: w960 -> [w982 w1033]
              tunnel: [w981 w1032] -> w959
              tunnel: [w980 w1031] -> w958
              frame True {
                n432 = Greater?(x=w979, y=4.0) -> (0:w984:bool)
                n433 = case shown="True" w984 {
                  tunnel: w989 -> [w994 w1013]
                  tunnel: w988 -> [w995 w1012]
                  tunnel: w987 -> [w996 w1011]
                  tunnel: w986 -> [w999 w1010]
                  tunnel: [w994 w1006] -> w993
                  tunnel: [w995 w1007] -> w992
                  tunnel: [w996 w1009] -> w991
                  tunnel: [w1000 w1008] -> w990
                  tunnel: w979 -> [_ w1005]
                  tunnel: w983 -> [w997 w1004]
                  tunnel: w982 -> [w998 w1003]
                  tunnel: [w997 w1002] -> w981
                  tunnel: [w998 w1001] -> w980
                  frame False {
                    n434 = Increment(x=w999) -> (x+1=w1000:i32)
                  }
                  frame True {
                    n435 = Greater?(x=w1005, y=5.0) -> (0:w1014:bool)
                    n436 = case shown="True" w1014 {
                      tunnel: w1013 -> [w1022 w1029]
                      tunnel: w1012 -> [w1021 w1028]
                      tunnel: w1011 -> [w1019 w1027]
                      tunnel: w1010 -> [w1020 w1025]
                      tunnel: [w1022 w1029] -> w1006
                      tunnel: [w1021 w1028] -> w1007
                      tunnel: [w1019 w1027] -> w1009
                      tunnel: [w1020 w1025] -> w1008
                      tunnel: w1004 -> [w1018 w1026]
                      tunnel: w1003 -> [w1016 w1024]
                      tunnel: [w1017 w1026] -> w1002
                      tunnel: [w1016 w1023] -> w1001
                      frame False {
                        n437 = Increment(x=w1018) -> (x+1=w1017:i32)
                      }
                      frame True {
                        n438 = Increment(x=w1024) -> (x+1=w1023:i32)
                      }
                    }
                  }
                }
              }
              frame False {
                n439 = Greater?(x=w1030, y=1.0) -> (0:w1035:bool)
                n440 = case shown="True" w1035 {
                  tunnel: w1040 -> [w1046 w1064]
                  tunnel: w1039 -> [w1048 w1063]
                  tunnel: w1038 -> [w1049 w1062]
                  tunnel: w1037 -> [w1047 w1061]
                  tunnel: [w1045 w1057] -> w1044
                  tunnel: [w1048 w1058] -> w1043
                  tunnel: [w1049 w1060] -> w1042
                  tunnel: [w1047 w1059] -> w1041
                  tunnel: w1030 -> [_ w1056]
                  tunnel: w1034 -> [w1050 w1055]
                  tunnel: w1033 -> [w1051 w1054]
                  tunnel: [w1050 w1053] -> w1032
                  tunnel: [w1051 w1052] -> w1031
                  frame False {
                    n441 = Increment(x=w1046) -> (x+1=w1045:i32)
                  }
                  frame True {
                    n442 = Greater?(x=w1056, y=2.0) -> (0:w1065:bool)
                    n443 = case shown="False" w1065 {
                      tunnel: w1064 -> [w1073 w1080]
                      tunnel: w1063 -> [w1068 w1079]
                      tunnel: w1062 -> [w1071 w1074]
                      tunnel: w1061 -> [w1072 w1077]
                      tunnel: [w1073 w1080] -> w1057
                      tunnel: [w1067 w1079] -> w1058
                      tunnel: [w1071 w1075] -> w1060
                      tunnel: [w1072 w1077] -> w1059
                      tunnel: w1055 -> [w1069 w1078]
                      tunnel: w1054 -> [w1070 w1076]
                      tunnel: [w1069 w1078] -> w1053
                      tunnel: [w1070 w1076] -> w1052
                      frame False {
                        n444 = Increment(x=w1068) -> (x+1=w1067:i32)
                      }
                      frame True {
                        n445 = Increment(x=w1074) -> (x+1=w1075:i32)
                      }
                    }
                  }
                }
              }
            }
            n446 = call-poly <vilib>:"DAQmx Create Virtual Channel.vi"("lines"=tag "Dev1/port0/line0") -> ("task out"=w977:refnum<k21>)  [unwired: 13 in, 1 out]
            n447 = call <vilib>:"DAQmx Start Task.vi"("task/channels in"=w977) -> ("task out"=w976:refnum<k21>)  [unwired: 13 in, 1 out]
            n448 = call-poly <vilib>:"DAQmx Write.vi"("task/channels in"=w976, "data"=TRUE) -> ("task out"=w975:refnum<k21>)  [unwired: 11 in, 2 out]
            n449 = call <vilib>:"DAQmx Stop Task.vi"("task/channels in"=w975) -> ()  [unwired: 13 in, 2 out]
          }
        }
        n450 = Increment(x=w227) -> (x+1=w217:i32)
        "Trial" <- w217
        n451 = Divide(x=w217, y=w218) -> (x/y=→"Slide":dbl)
        "Stim 1" <- w204
        "Stim 2" <- w202
        "Stim 3" <- w200
        "Stim 4" <- w154
      }
    }
    frame #3 {
      n452 = Close File(refnum=w1087) -> ()  [unwired: 1 in, 2 out]
      n453 = Close File(refnum=w1081) -> ()  [unwired: 1 in, 2 out]
      n454 = call-poly <vilib>:"DAQmx Create Virtual Channel.vi"("physical channels"=tag "Dev1/ao1") -> ("task out"=w1090:refnum<k21>)  [unwired: 13 in, 1 out]
      n455 = call-poly <vilib>:"DAQmx Create Virtual Channel.vi"("physical channels"=tag "Dev1/ao0") -> ("task out"=w1084:refnum<k21>)  [unwired: 13 in, 1 out]
      n456 = call <vilib>:"DAQmx Start Task.vi"("task/channels in"=w1090) -> ("task out"=w1092:refnum<k21>)  [unwired: 13 in, 1 out]
      n457 = call <vilib>:"DAQmx Start Task.vi"("task/channels in"=w1084) -> ("task out"=w1086:refnum<k21>)  [unwired: 13 in, 1 out]
      n458 = call-poly <vilib>:"DAQmx Write.vi"("task/channels in"=w1092, "data"=5.0) -> ("task out"=w1091:refnum<k21>)  [unwired: 11 in, 2 out]
      n459 = call-poly <vilib>:"DAQmx Write.vi"("task/channels in"=w1086, "data"=5.0) -> ("task out"=w1085:refnum<k21>)  [unwired: 11 in, 2 out]
      n460 = call <vilib>:"DAQmx Stop Task.vi"("task/channels in"=w1091) -> ()  [unwired: 13 in, 2 out]
      n461 = call <vilib>:"DAQmx Stop Task.vi"("task/channels in"=w1085) -> ()  [unwired: 13 in, 2 out]
    }
  }
